vi "Enable UI Elements.vi"(6 "Disabled":T1(ring), 11 "Car Wash Console in":refnum<class "Car Wash Console.lvclass">) -> (3 "Car Wash Console out":refnum<class "Car Wash Console.lvclass">)   [LabVIEW 2016, in "CLD Exam - Car Wash.lvlib" / "Car Wash Console.lvclass"]
uses:
  Car Wash Console.lvclass
  Car Wash Console.lvclass/Car Wash Console.ctl
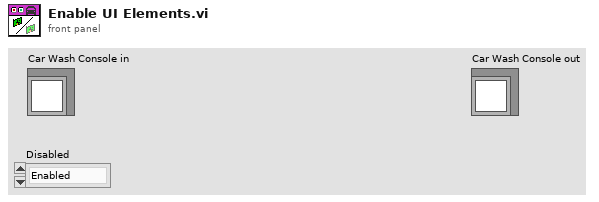
[diagram p1: front panel]
types:
  T1 = enum8{"Enabled", "Disabled", "Disabled and Grayed Out"}
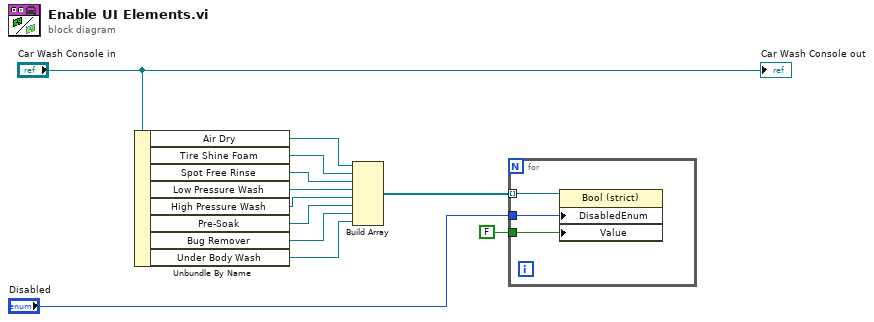
[diagram p0: block diagram]
diagram:
  n1 = Unbundle By Name("Car Wash Console in") -> ("Air Dry"=w11:refnum<vi>, "Tire Shine Foam"=w10:refnum<vi>, "Spot Free Rinse"=w9:refnum<vi>, "Low Pressure Wash"=w8:refnum<vi>, "High Pressure Wash"=w7:refnum<vi>, "Pre-Soak"=w6:refnum<vi>, "Bug Remover"=w5:refnum<vi>, "Under Body Wash"=w4:refnum<vi>)
  n2 = Build Array(w11, w10, w9, w8, w7, w6, w5, w4) -> (w3:refnum<vi>[])
  n3 = for {
    tunnel: "Disabled" -> [w15]
    tunnel: w3 -> [w14] mode=indexing
    tunnel: FALSE -> [w13]
    n4 = property class="Bool (strict)"(reference=w14, "DisabledEnum"=w15, "Value"=w13) -> ()  [unwired: 1 in, 2 out]
  }
  "Car Wash Console out" <- "Car Wash Console in"
